vi "HornReceipe_Local_Read_INI_Sub_VI.vi"(11 "Config File Path":path) -> (3 "output cluster":T1)   [LabVIEW 2017]
uses:
  <vilib>/Utility/config.llb/Read Key (I32).vi
  <vilib>/Utility/config.llb/Read Key (Double).vi
  <vilib>/Utility/config.llb/Read Key (String).vi
  <vilib>/Utility/config.llb/Read Key (Path).vi
  <vilib>/Utility/config.llb/NI_LVConfig.lvlib
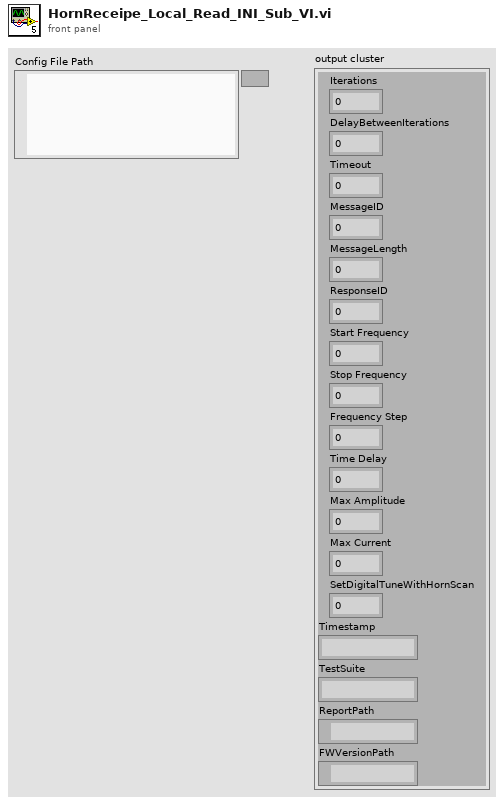
[diagram p1: front panel]
types:
  T1 = cluster{"Iterations":u64, "DelayBetweenIterations":u32, "Timeout":u32, "MessageID":u32, "MessageLength":u32, "ResponseID":i32, "Start Frequency":u32, "Stop Frequency":u32, "Frequency Step":u16, "Time Delay":u16, "Max Amplitude":u16, "Max Current":u16, "SetDigitalTuneWithHornScan":u16, "Timestamp":string, "TestSuite":string, "ReportPath":path, "FWVersionPath":path}
  T2 = typedef "NI_LVConfig.lvlib/Config Data RefNum.ctl" = refnum<k1>
  T3 = cluster{u64, u32, u32, i32, i32, i32, i32, i32, i16, dbl, i16, i16, i16, "value":string, "value":string, "value":path, path}
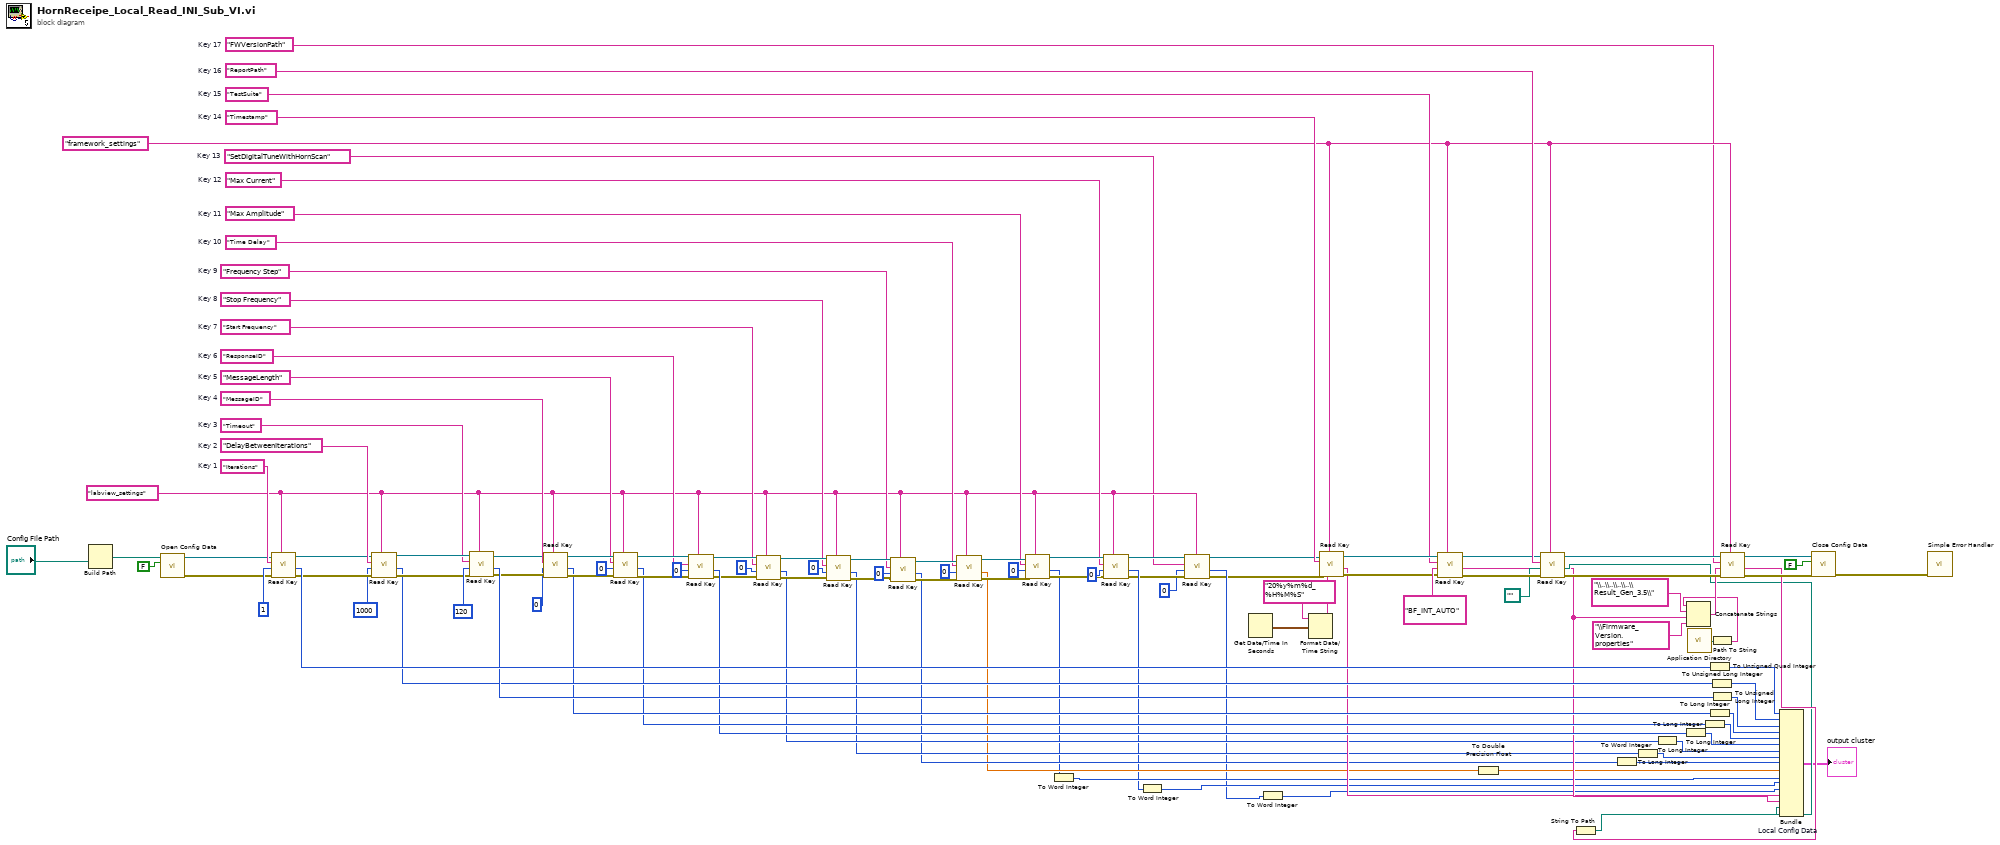
[diagram p0: block diagram]
diagram:
  w3 = "SetDigitalTuneWithHornScan"  # Key 13
  w36 = "Max Current"  # Key 12
  w37 = "Max Amplitude"  # Key 11
  w38 = "Time Delay"  # Key 10
  w39 = "Frequency Step"  # Key 9
  w40 = "Stop Frequency"  # Key 8
  w41 = "Start Frequency"  # Key 7
  w57 = "ResponseID"  # Key 6
  w58 = "MessageLength"  # Key 5
  w70 = "MessageID"  # Key 4
  w80 = "FWVersionPath"  # Key 17
  w92 = "Timestamp"  # Key 14
  w87 = "TestSuite"  # Key 15
  w93 = "Timeout"  # Key 3
  w102 = "ReportPath"  # Key 16
  w107 = "DelayBetweenIterations"  # Key 2
  w109 = "Iterations"  # Key 1
  w81 = "framework_settings" ("section")
  w4 = "labview_settings" ("section")
  n1 = Build Path(name or relative path="Config File Path") -> (appended path=w111:path)  [unwired: 1 in]
  n2 = call <vilib>:"Open Config Data.vi"("create file if necessary (T)"=FALSE ("create file if necessary? (T)"), "configuration file path"=w111) -> ("error out"=w73:errorcluster, "refnum"=w72:T2)  [unwired: 7 in, 1 out]
  n3 = call-poly <vilib>:"Read Key.vi"("section"=w4, "error in (no error)"=w73, "default value"=1, "key"=w109, "refnum"=w72) -> ("error out"=w105:errorcluster, "value"=w108:i32, "refnum out"=w106:T2)  [unwired: 4 out]
  n4 = call-poly <vilib>:"Read Key.vi"("section"=w4, "error in (no error)"=w105, "default value"=1000, "key"=w107, "refnum"=w106) -> ("error out"=w100:errorcluster, "value"=w71:i32, "refnum out"=w99:T2)  [unwired: 4 out]
  n5 = call-poly <vilib>:"Read Key.vi"("section"=w4, "error in (no error)"=w100, "default value"=120, "key"=w93, "refnum"=w99) -> ("error out"=w66:errorcluster, "value"=w97:i32, "refnum out"=w69:T2)  [unwired: 4 out]
  n6 = call-poly <vilib>:"Read Key.vi"("section"=w4, "error in (no error)"=w66, "default value"=0, "key"=w70, "refnum"=w69) -> ("error out"=w64:errorcluster, "value"=w63:i32, "refnum out"=w68:T2)  [unwired: 4 out]
  n7 = call-poly <vilib>:"Read Key.vi"("section"=w4, "error in (no error)"=w64, "default value"=0, "key"=w58, "refnum"=w68) -> ("error out"=w65:errorcluster, "value"=w60:i32, "refnum out"=w67:T2)  [unwired: 4 out]
  n8 = call-poly <vilib>:"Read Key.vi"("section"=w4, "error in (no error)"=w65, "default value"=0, "key"=w57, "refnum"=w67) -> ("error out"=w31:errorcluster, "value"=w59:i32, "refnum out"=w47:T2)  [unwired: 4 out]
  n9 = call-poly <vilib>:"Read Key.vi"("section"=w4, "error in (no error)"=w31, "default value"=0, "key"=w41, "refnum"=w47) -> ("error out"=w27:errorcluster, "value"=w22:i32, "refnum out"=w46:T2)  [unwired: 4 out]
  n10 = call-poly <vilib>:"Read Key.vi"("section"=w4, "error in (no error)"=w27, "default value"=0, "key"=w40, "refnum"=w46) -> ("error out"=w30:errorcluster, "value"=w20:i32, "refnum out"=w45:T2)  [unwired: 4 out]
  n11 = call-poly <vilib>:"Read Key.vi"("section"=w4, "error in (no error)"=w30, "default value"=0, "key"=w39, "refnum"=w45) -> ("error out"=w29:errorcluster, "value"=w18:i32, "refnum out"=w44:T2)  [unwired: 4 out]
  n12 = call-poly <vilib>:"Read Key.vi"("section"=w4, "error in (no error)"=w29, "default value"=0, "key"=w38, "refnum"=w44) -> ("error out"=w26:errorcluster, "value"=w16:dbl, "refnum out"=w43:T2)  [unwired: 4 out]
  n13 = call-poly <vilib>:"Read Key.vi"("section"=w4, "error in (no error)"=w26, "default value"=0, "key"=w37, "refnum"=w43) -> ("error out"=w28:errorcluster, "value"=w14:i32, "refnum out"=w42:T2)  [unwired: 4 out]
  n14 = To Word Integer(number=w14) -> (16bit integer=w13:i16)
  n15 = call-poly <vilib>:"Read Key.vi"("section"=w4, "error in (no error)"=w28, "default value"=0, "key"=w36, "refnum"=w42) -> ("error out"=w7:errorcluster, "value"=w12:i32, "refnum out"=w9:T2)  [unwired: 4 out]
  n16 = To Word Integer(number=w12) -> (16bit integer=w11:i16)
  n17 = call-poly <vilib>:"Read Key.vi"("section"=w4, "error in (no error)"=w7, "default value"=0, "key"=w3, "refnum"=w9) -> ("error out"=w6:errorcluster, "value"=w10:i32, "refnum out"=w8:T2)  [unwired: 4 out]
  n18 = Get Date/Time In Seconds() -> (seconds since 1Jan1904=w94:timestamp)
  n19 = To Word Integer(number=w10) -> (16bit integer=w2:i16)
  n20 = Format Date/Time String(time format string (%c)="20%y%m%d_%H%M%S", seconds (now)=w94) -> (date/time string=w95:string)  [unwired: 1 out]
  n21 = call-poly <vilib>:"Read Key.vi"("section"=w81, "error in (no error)"=w6, "default value"=w95, "key"=w92, "refnum"=w8) -> ("error out"=w89:errorcluster, "value"=w32:string, "refnum out"=w90:T2)  [unwired: 1 in, 3 out]
  n22 = call-poly <vilib>:"Read Key.vi"("section"=w81, "error in (no error)"=w89, "default value"="BF_INT_AUTO", "key"=w87, "refnum"=w90) -> ("error out"=w88:errorcluster, "value"=w33:string, "refnum out"=w91:T2)  [unwired: 1 in, 3 out]
  n23 = To Double Precision Float(number=w16) -> (double precision float=w15:dbl)
  n24 = call-poly <vilib>:"Read Key.vi"("section"=w81, "error in (no error)"=w88, "default value"=path "", "key"=w102, "refnum"=w91) -> ("error out"=w82:errorcluster, "value"=w34:path, "refnum out"=w85:T2)  [unwired: 1 in, 3 out]
  n25 = To Word Integer(number=w18) -> (16bit integer=w17:i16)
  n26 = To Long Integer(number=w20) -> (32bit integer=w19:i32)
  n27 = To Long Integer(number=w22) -> (32bit integer=w21:i32)
  n28 = To Long Integer(number=w59) -> (32bit integer=w25:i32)
  n29 = call <vilib>:"Application Directory.vi"() -> ("Application Directory"=w76:path)
  n30 = To Long Integer(number=w60) -> (32bit integer=w61:i32)
  n31 = To Unsigned Quad Integer(1:w108) -> (0:w115:u64)
  n32 = To Long Integer(number=w63) -> (32bit integer=w62:i32)
  n33 = To Unsigned Long Integer(number=w71) -> (unsigned 32bit integer=w24:u32)
  n34 = Path To String(path=w76) -> (string=w75:string)
  n35 = Concatenate Strings(w75, "\\..\\..\\..\\..\\Result_Gen_3.5\\" ("default value"), w33, "\\Firmware_Version.properties" ("default value")) -> (w79:string)
  n36 = To Unsigned Long Integer(number=w97) -> (unsigned 32bit integer=w23:u32)
  n37 = call-poly <vilib>:"Read Key.vi"("section"=w81, "error in (no error)"=w82, "default value"=w79, "key"=w80, "refnum"=w85) -> ("error out"=w83:errorcluster, "value"=w74:string, "refnum out"=w84:T2)  [unwired: 1 in, 3 out]
  n38 = String To Path(string=w74) -> (path=w35:path)
  n39 = Bundle "Local Config Data"(w115, w24, w23, w62, w61, w25, w21, w19, w17, w15, w13, w11, w2, "value"=w32, "value"=w33, "value"=w34, w35) -> (→"output cluster":T3)  [unwired: 1 in]
  n40 = call <vilib>:"Close Config Data.vi"("error in (no error)"=w83, "write file if changed (T)"=FALSE ("write configuration file? (T)"), "refnum"=w84) -> ("error out"=w112:errorcluster)  [unwired: 8 out]
  n41 = call <vilib>:"Simple Error Handler.vi"("error in (no error)"=w112) -> ()  [unwired: 1 in, 8 out]
